vi "add_killOcc.vi"(0 "Host_Reference":refnum<class "HGF_Reference.lvclass">, 2 "timeout in ms (-1)":i32, 5 "error in (no error)":errorcluster, 7 "ID":string, 9 "killNotifier":refnum<notifier>) -> (14 "dup Host_Reference":refnum<class "HGF_Reference.lvclass">, 16 "dup timeout in ms (-1)":i32, 19 "error out":errorcluster)   [LabVIEW 2009, in "MoAgSy.lvlib" / "MoAgSy_Host.lvclass"]
doc: "<B>public</B> VI adds kill occurence to referenced Host.\nKill Occurrences are used to stop a running agent immediately.\n\nF.Berck@gsi.de\nGSI Darmstadt 2009"
uses:
  MoAgSy_Host.lvclass
  HGF_BaseClasses/HGF_Reference/HGF_Reference.lvclass
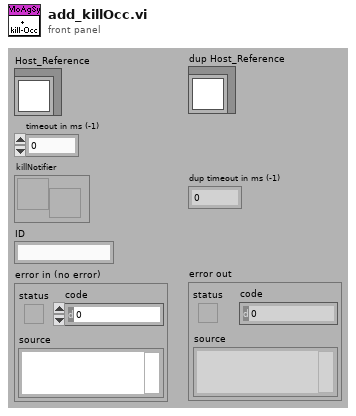
[diagram p1: front panel]
types:
  T1 = cluster{"killNotifier":refnum<notifier>, "Agent ID":string}
  T2 = cluster{"killNotifier":refnum<notifier>, "Agent ID":string}[]
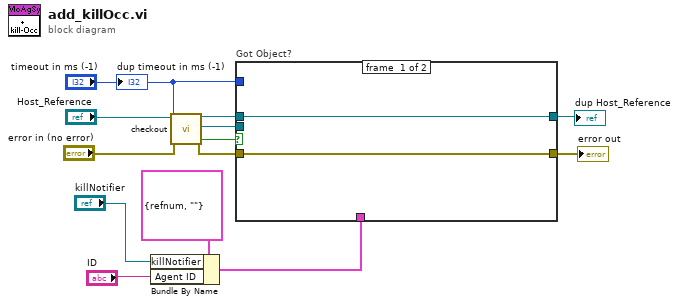
[diagram p0: block diagram]
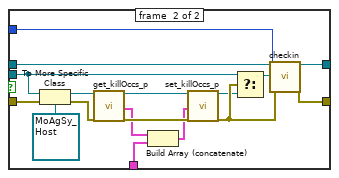
[diagram p2: hidden frame]
diagram:
  n1 = Bundle By Name(cluster=T1 {"killNotifier"=refnum, "Agent ID"=""} ("Kill Occ"), "killNotifier"="killNotifier", "Agent ID"="ID") -> (w2:T1)
  n2 = call "checkout.vi"("HGF_Reference"="Host_Reference", "timeout in ms (-1)"="timeout in ms (-1)", "error in (no error)"="error in (no error)") -> ("dup HGF_Reference"=w10:refnum<class "HGF_Reference.lvclass">, "Object"=w12:refnum<class>, "got object?"=w11:bool, "error out"=w13:errorcluster)  [unwired: 13 out]
  n3 = case "Got Object?" shown="True" w11 {
    tunnel: w12 -> [_ w26]
    tunnel: w10 -> [w15 w31]
    tunnel: [w15 w30] -> w7
    tunnel: "timeout in ms (-1)" -> [_ w29]
    tunnel: [w14 w28] -> w6
    tunnel: w13 -> [w14 w27]
    tunnel: w2 -> [_ w16]
    frame #0 {
    }
    frame #1 {
      n4 = To More Specific Class(target class=refnum<class "MoAgSy_Host.lvclass"> refnum ("MoAgSy.lvlib:MoAgSy_Host.lvclass"), reference=w26, error in=w27) -> (specific class reference=w24:refnum<class "MoAgSy_Host.lvclass">, error out=w23:errorcluster)
      n5 = call "get_killOccs_p.vi"("MoAgSy_Host"=w24, "error in (no error)"=w23) -> ("dup MoAgSy_Host"=w22:refnum<class "MoAgSy_Host.lvclass">, "Kill Occs"=w18:T2, "error out"=w21:errorcluster)  [unwired: 15 out]
      n6 = Build Array (concatenate)(w18, w16) -> (w17:T2)
      n7 = call "set_killOccs_p.vi"("MoAgSy_Host"=w22, "Kill Occs"=w17, "error in (no error)"=w21) -> ("dup MoAgSy_Host"=w19:refnum<class "MoAgSy_Host.lvclass">, "error out"=w20:errorcluster)  [unwired: 1 in, 14 out]
      n8 = Select(t=w26, s=w20, f=w19) -> (s? t:f=w25:refnum<class>)
      n9 = call "checkin.vi"("HGF_Reference"=w31, "Object"=w25, "timeout /ms (-1)"=w29, "error in (no error)"=w20) -> ("dup HGF_Reference"=w30:refnum<class "HGF_Reference.lvclass">, "error out"=w28:errorcluster)  [unwired: 14 out]
    }
  }
  "dup Host_Reference" <- w7
  "error out" <- w6
  "dup timeout in ms (-1)" <- "timeout in ms (-1)"
